vi "set position.vi"(8 "error in (no error)":errorcluster, 9 "Microsteps":i32, 10 "Device Number":i8, 11 "VISA resource name":refnum<visa-resource-name>) -> (0 "error out":errorcluster)   [LabVIEW 2020]
uses:
  Public/Utility/Request.ctl
  ZaberTSeries.lvlib
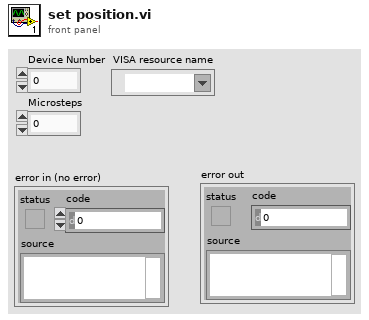
[diagram p1: front panel]
types:
  T1 = typedef "ZaberTSeries.lvlib/Request.ctl" = cluster{"Device Number":u8, "Command":u8, "Data":i32, "Response Count":i32}
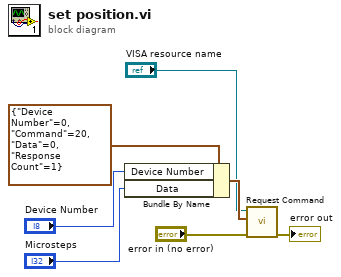
[diagram p0: block diagram]
diagram:
  n1 = Bundle By Name(cluster=T1 {"Device Number"=0, "Command"=20, "Data"=0, "Response Count"=1} ("Request"), "Device Number"="Device Number", "Data"="Microsteps") -> (w6:T1)
  n2 = call "Request Command.vi"("error in (no error)"="error in (no error)", "Request"=w6, "VISA resource name"="VISA resource name") -> ("error out"=→"error out":errorcluster)  [unwired: 5 in, 3 out]
